vi "error custom defs.vi"(1 "error in (no error)":errorcluster) -> (0 "error out":errorcluster)   [LabVIEW 2010, in "ErrorLog.lvlib"]
uses:
  ErrorLog.lvlib
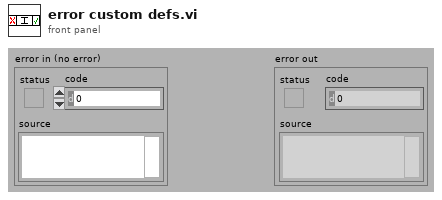
[diagram p1: front panel]
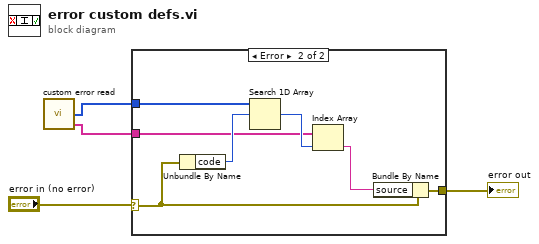
[diagram p0: block diagram]
diagram:
  n1 = call "custom error read.vi"() -> ("Description"=w1:string[], "Codes"=w2:i32[])  [unwired: 3 in, 1 out]
  n2 = case shown="Error" "error in (no error)" {
    selector: "error in (no error)" -> [w5 w9]
    tunnel: [w5 w10] -> w3
    tunnel: w2 -> [_ w7]
    tunnel: w1 -> [_ w6]
    frame No Error {
    }
    frame Error {
      n3 = Unbundle By Name(w9) -> ("code"=w12:i32)
      n4 = Search 1D Array(1D array=w7, element=w12) -> (index of element=w11:i32)  [unwired: 1 in]
      n5 = Index Array(array=w6, index=w11) -> (element=w8:string)
      n6 = Bundle By Name(cluster=w9, "source"=w8) -> (w10:errorcluster)
    }
  }
  "error out" <- w3
